vi "to string.vi"(8 "error in":errorcluster, 11 "Digitizer Channel configuration":refnum<class "Digitizer Channel configuration.lvclass">) -> (0 "error out":errorcluster, 1 "data":string, 2 "version":string, 3 "Digitizer Channel configuration out":refnum<class "Digitizer Channel configuration.lvclass">)   [LabVIEW 2025, in "Digitizer.lvlib" / "Digitizer Channel configuration.lvclass"]
doc: "Provides an interface for saving a module configuration to a file or other serialized data source. It is recommended that all children of this class store data in two sets--data required for its own initialization, and any data required for parent initialization--and that each implementation uses the <b>Call Parent Method</b> primitive to serialize parent information.Copyright 2017 National Instruments Corporation\n\nLicensed under the Apache License, Version 2.0 (the \"License\"); you may not use this file except in compliance with the License. You may obtain a copy of the License at http://www.apache.org/licenses/LICENSE-2.0\nUnless required by applicable law or agreed to in writing, software distributed under the License is distributed on an \"AS IS\" BASIS, WITHOUT WARRANTIES OR CONDITIONS OF ANY KIND, either express or implied. See the License for the specific language governing permissions and limitations under the License."
uses:
  Digitizer Channel configuration.lvclass
  Digitizer Channel configuration.lvclass/Digitizer Channel configuration.ctl
  Users/Public/Documents/Sandia National Labs/TSS Plugin/Abstract Engine.lvlibp/Plugin/Abstract/Channel configuration/Channel configuration.lvclass
  Users/Public/Documents/Sandia National Labs/TSS Plugin/CEF.lvlibp/serializable configuration/CEF_serializable configuration.lvclass
  Users/Public/Documents/Sandia National Labs/TSS Plugin/CEF.lvlibp
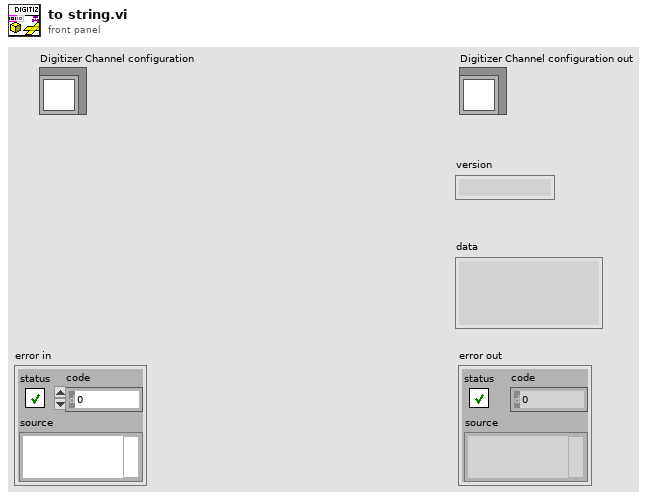
[diagram p1: front panel]
types:
  T1 = typedef "Digitizer.lvlib/Digitizer Channel configuration.lvclass/Digitizer Channel Setting.ctl" = cluster{"Max":dbl, "Min":dbl, "Data Reduction":string, "Averging Points":u32, "Decimate Interval":u32, "Aperture Options":cluster{"Tolerance":u32, "Burst":u32, "Min SampleRate":u32, "Min SampleIndex":u32}}
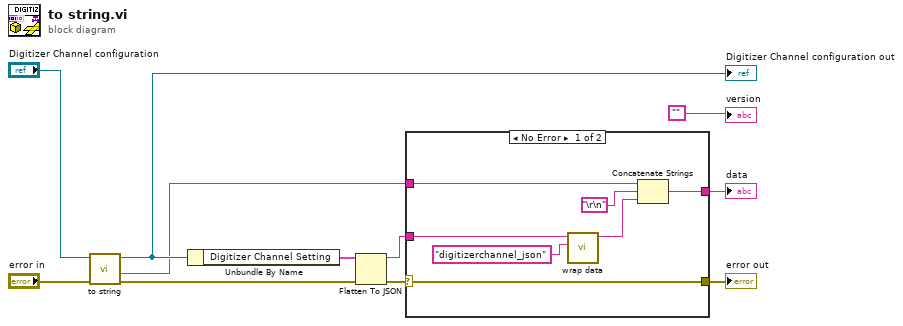
[diagram p0: block diagram]
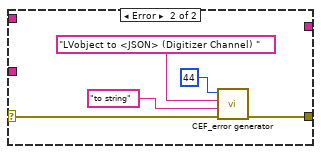
[diagram p2: hidden frame]
diagram:
  n1 = call-parent "to string.vi"("error in"="error in", "Channel configuration"="Digitizer Channel configuration") -> ("error out"=w10:errorcluster, "data"=w2:string, "Channel configuration out"=w7:refnum<class "Digitizer Channel configuration.lvclass">)  [unwired: 6 in, 1 out]
  "Digitizer Channel configuration out" <- w7
  n2 = Unbundle By Name(w7) -> ("Digitizer Channel Setting"=w11:T1)
  n3 = Flatten To JSON(anything=w11, error in (no error)=w10) -> (JSON string=w3:string, 11:w6:errorcluster)  [unwired: 1 in]
  n4 = case shown="No Error" w6 {
    selector: w6 -> [w18 w20]
    tunnel: [w18 w19] -> w5
    tunnel: w3 -> [w15 _]
    tunnel: w2 -> [w14 _]
    tunnel: [w12 _] -> w4
    frame No Error {
      n5 = call "wrap data.vi"("identifier"="digitizerchannel_json" ("additional identifier"), "data to wrap"=w15) -> ("wrapped data"=w17:string)  [unwired: 9 in]
      n6 = Concatenate Strings(w14, "\r\n", w17) -> (w12:string)
    }
    frame Error {
      n7 = call "CEF_error generator.vi"("error in"=w20, "source"="to string" ("message"), "append error message"="LVobject to <JSON> (Digitizer Channel) " ("message"), "error code (0)"=44) -> ("error out"=w19:errorcluster)  [unwired: 5 in]
    }
  }
  "error out" <- w5
  "data" <- w4
  "version" <- ""
